vi "command.vi"(6 "timeout ms (1000)":i32=1000, 8 "error in (no error)":errorcluster, 10 "Query":string, 11 "TCP in":refnum<k5>) -> (0 "error out":errorcluster, 3 "TCP out":refnum<k5>)   [LabVIEW 2025, in "Newtons4thEkg.lvlib"]
uses:
  Newtons4thEkg.lvlib
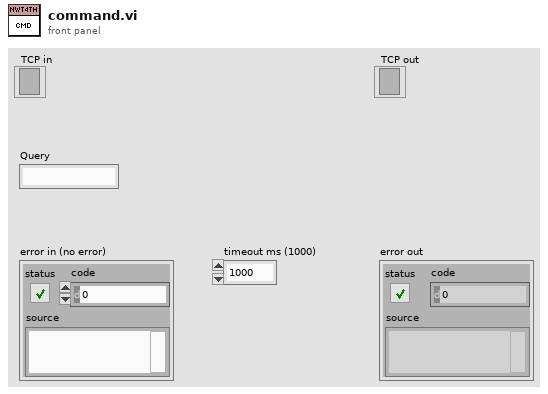
[diagram p1: front panel]
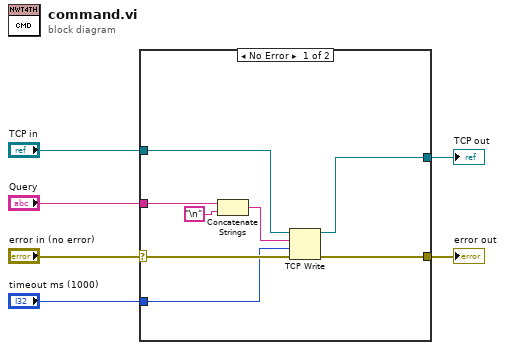
[diagram p0: block diagram]
diagram:
  n1 = case shown="No Error" "error in (no error)" {
    selector: "error in (no error)" -> [w11 w16]
    tunnel: "Query" -> [w14 _]
    tunnel: "TCP in" -> [w10 w15]
    tunnel: "timeout ms (1000)" -> [w7 _]
    tunnel: [w8 w16] -> w2
    tunnel: [w9 w15] -> w1
    frame No Error {
      n2 = Concatenate Strings(w14, "\n") -> (w12:string)
      n3 = TCP Write(connection ID=w10, data in=w12, error in (no error)=w11, 9:w7) -> (connection ID out=w9:refnum<k5>, error out=w8:errorcluster)  [unwired: 1 out]
    }
    frame Error {
    }
  }
  "TCP out" <- w1
  "error out" <- w2
